vi "Read ADU Packet.vi"(8 "error in":errorcluster, 10 "Network Protocol":refnum<class "Network Protocol.lvclass">, 11 "ASCII transmission data unit in":refnum<class "ASCII Data Unit.lvclass">) -> (0 "error out":errorcluster, 1 "modbus data unit":refnum<class "Modbus Data Unit (PDU).lvclass">, 2 "Network Protocol out":refnum<class "Network Protocol.lvclass">, 3 "ASCII transmission data unit out":refnum<class "ASCII Data Unit.lvclass">, 5 "PDU Valid?":bool)   [LabVIEW 2020, in "SubVIs.lvlib" / "ASCII Data Unit.lvclass"]
uses:
  <vilib>/Modbus/subvis/Transmission Data Unit (ADU)/ASCII Data Unit/ASCII Data Unit.lvclass
  C:/builds/penguin/iak/lvdsc/trunk/20.0/lv/vi.lib/Modbus/subvis/Transmission Data Unit (ADU)/Transmission Data Unit/Transmission Data Unit.lvclass
  <vilib>/Modbus/subvis/Modbus Data Unit (PDU)/Modbus Data Unit (PDU).lvclass
  <vilib>/Modbus/subvis/Protocol/Interfaces/Network Protocol/Network Protocol.lvclass
  <vilib>/Modbus/subvis/Protocol/Serial/Serial Slave/Serial Slave.lvclass
  <vilib>/Modbus/subvis/Protocol/Serial/Serial Slave/Serial Slave.lvclass/Serial Slave.ctl
  <vilib>/Modbus/subvis/Protocol/Serial/Serial Master/Serial Master.lvclass
  <vilib>/Modbus/subvis/Protocol/Serial/Serial Master/Serial Master.lvclass/Serial Master.ctl
  <vilib>/Modbus/subvis/Transmission Data Unit (ADU)/Transmission Data Unit/Transmission Data Unit.lvclass/Transmission Data Unit.ctl
  <vilib>/Modbus/subvis/Modbus Data Unit (PDU)/Modbus Data Unit (PDU).lvclass/Modbus Data Unit (PDU).ctl
  <vilib>/Modbus/subvis/Transmission Data Unit (ADU)/ASCII Data Unit/ASCII Data Unit.lvclass/ASCII Data Unit.ctl
  <vilib>/ErrorRing/Error Ring.xnode
  <vilib>/Modbus/subvis/Transmission Data Unit (ADU)/Transmission Data Unit/Transmission Data Unit.lvclass
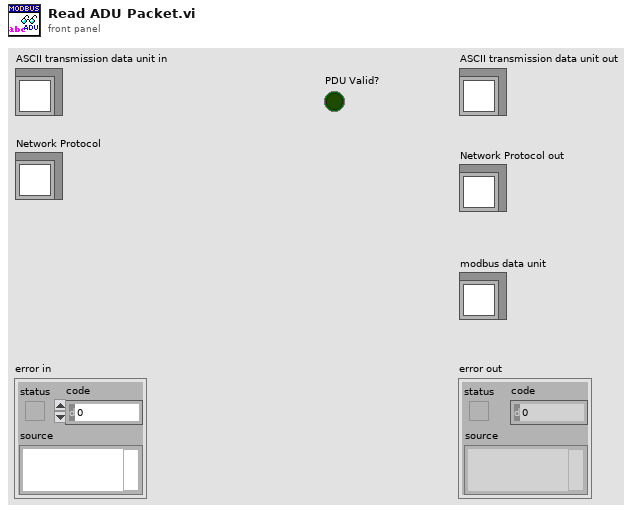
[diagram p1: front panel]
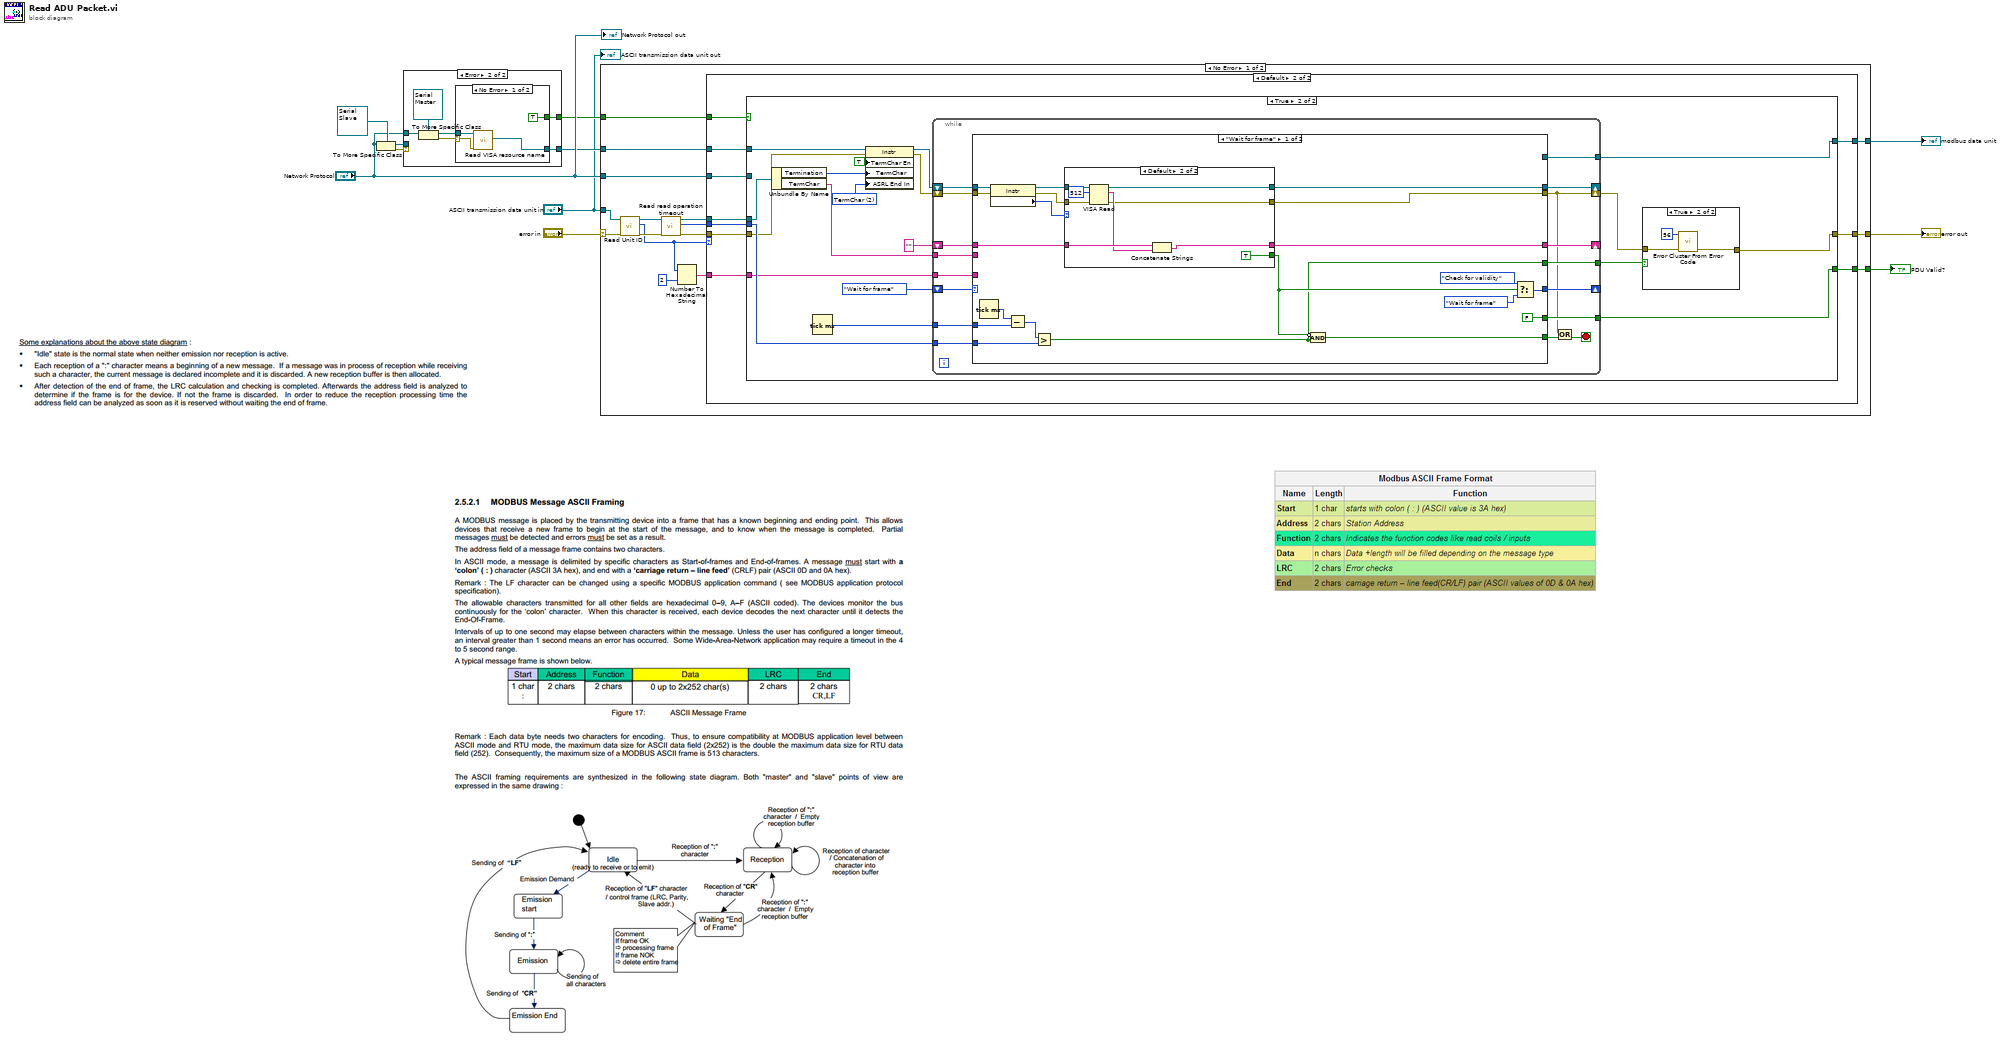
[diagram p0: block diagram]
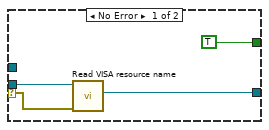
[diagram p2: hidden frame]
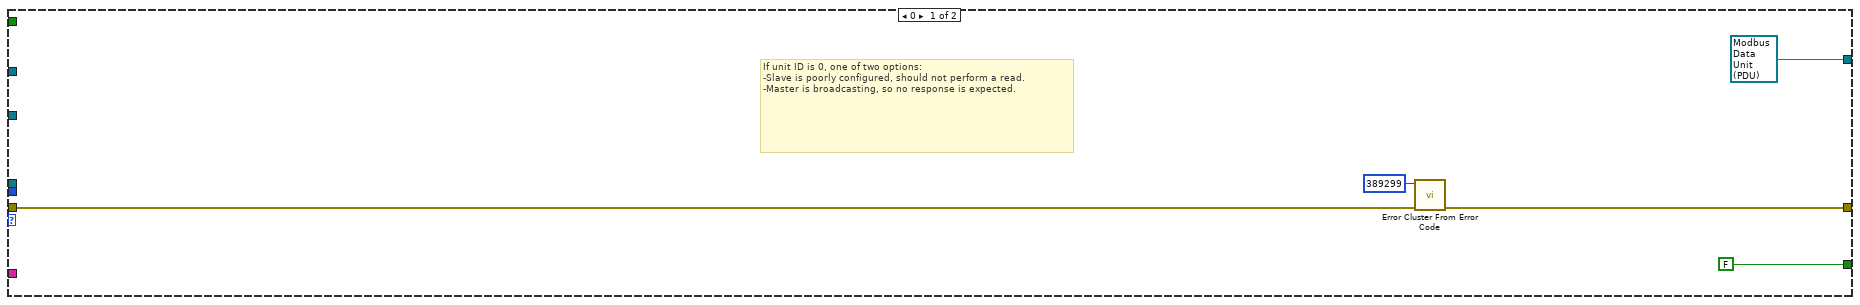
[diagram p4: hidden frame]
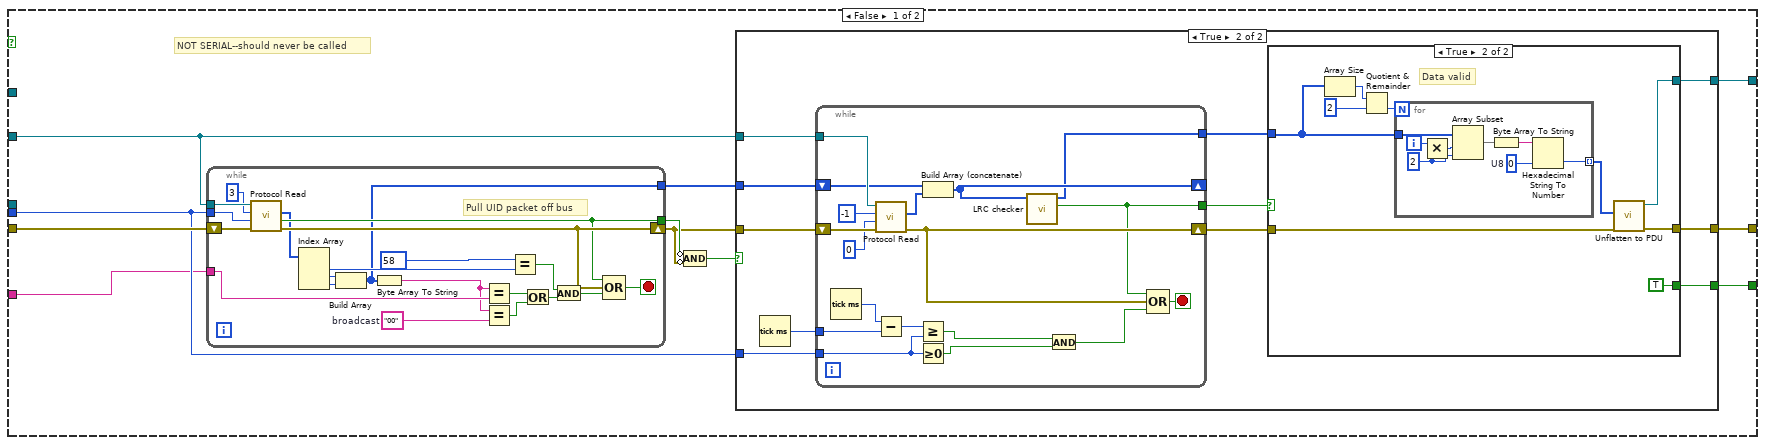
[diagram p5: hidden frame]
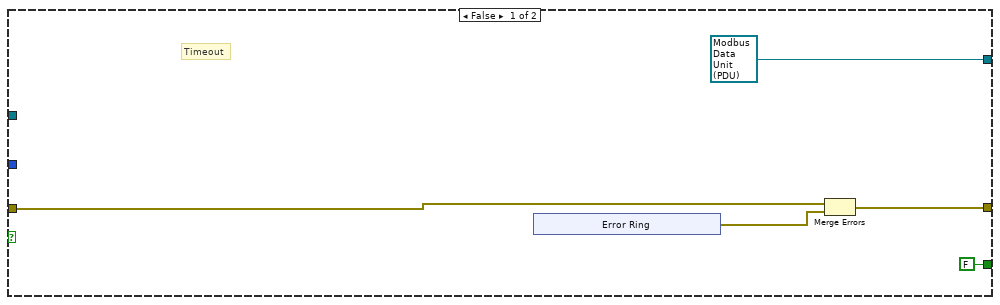
[diagram p6: hidden frame]
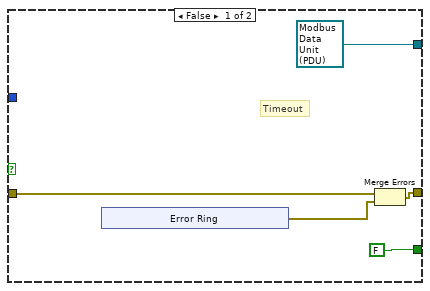
[diagram p7: hidden frame]
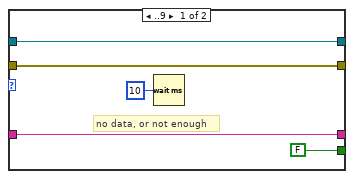
[diagram p9: hidden frame]
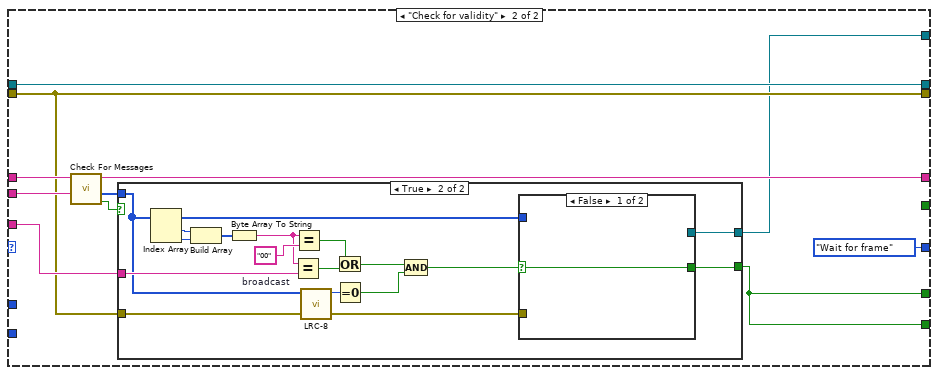
[diagram p10: hidden frame]
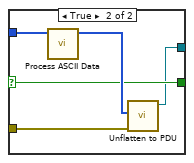
[diagram p12: hidden frame]
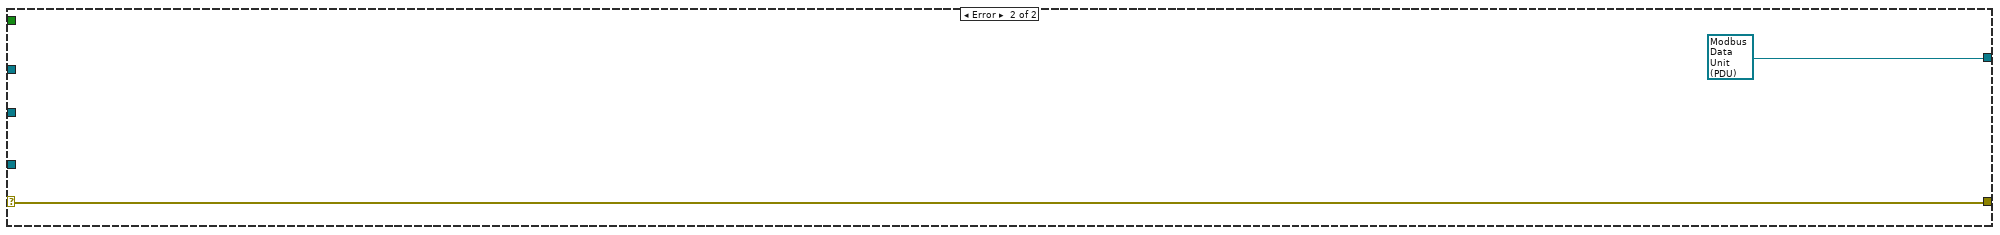
[diagram p13: hidden frame]
diagram:
  n1 = To More Specific Class(target class=refnum<class "Serial Slave.lvclass"> refnum ("Serial Master"), reference="Network Protocol") -> (specific class reference=w3:refnum<class "Serial Slave.lvclass">, error out=w6:errorcluster)  [unwired: 1 in]
  n2 = case shown="Error" w6 {
    selector: w6 -> [w13 _]
    tunnel: "Network Protocol" -> [_ w21]
    tunnel: [TRUE w18] -> w4
    tunnel: w3 -> [w14 _]
    tunnel: [w12 w16] -> w2
    frame No Error {
      n3 = call <vilib>:"Read VISA resource name.vi"("error in (no error)"=w13, "serial slave in"=w14) -> ("VISA resource name"=w12:refnum<visa-resource-name>)  [unwired: 7 in, 2 out]
    }
    frame Error {
      n4 = To More Specific Class(target class=refnum<class "Serial Master.lvclass"> refnum ("Serial Slave"), reference=w21) -> (specific class reference=w17:refnum<class "Serial Master.lvclass">, error out=w19:errorcluster)  [unwired: 1 in]
      n5 = case shown="No Error" w19 {
        selector: w19 -> [w23 _]
        tunnel: [TRUE _] -> w18
        tunnel: w17 -> [w24 _]
        tunnel: [w22 _] -> w16
        frame No Error {
          n6 = call <vilib>:"Read VISA resource name.vi"("error in (no error)"=w23, "serial master in"=w24) -> ("VISA resource name"=w22:refnum<visa-resource-name>)  [unwired: 7 in, 2 out]
        }
        frame Error {
        }
      }
    }
  }
  n7 = case shown="No Error" "error in" {
    selector: "error in" -> [w37 w262]
    tunnel: [w41 w262] -> w9
    tunnel: "ASCII transmission data unit in" -> [w27 _]
    tunnel: "Network Protocol" -> [w39 _]
    tunnel: [w40 refnum<class "Modbus Data Unit (PDU).lvclass"> refnum ("modbus data unit")] -> w10
    tunnel: [w33 _] -> w8
    tunnel: w4 -> [w32 _]
    tunnel: w2 -> [w28 _]
    frame No Error {
      n8 = call <vilib>:"Read Unit ID.vi"("error in"=w37, "transmission data unit in"=w27) -> ("error out"=w36:errorcluster, "unit ID"=w30:u8, "transmission data unit out"=w38:refnum<class "ASCII Data Unit.lvclass">)  [unwired: 7 in]
      n9 = call <vilib>:"Read read operation timeout.vi"("error in (no error)"=w36, "transmission data unit in"=w38) -> ("error out"=w35:errorcluster, "read operation timeout"=w34:i32, "transmission data unit out"=w26:refnum<class "ASCII Data Unit.lvclass">)  [unwired: 7 in]
      n10 = Number To Hexadecimal String(1:i16 2 ("width (-)"), 2:w30) -> (0:w29:string)
      n11 = case shown="Default" w30 {
        tunnel: w35 -> [w46 w52]
        tunnel: [w43 w56] -> w41
        tunnel: [refnum<class "Modbus Data Unit (PDU).lvclass"> refnum ("modbus data unit out") w55] -> w40
        tunnel: w39 -> [_ w51]
        tunnel: w34 -> [_ w54]
        tunnel: [FALSE w53] -> w33
        tunnel: w32 -> [_ w50]
        tunnel: w29 -> [_ w49]
        tunnel: w28 -> [_ w48]
        tunnel: w26 -> [_ w47]
        frame 0 {
          # "If unit ID is 0, one of two options:\n-Slave is poorly configured, should not perform a read.\n-Master is broadcasting, so no response is expected."
          n12 = call <vilib>:"Error Cluster From Error Code.vi"("error in (no error)"=w46, "error code (0)"=389299) -> ("error out"=w43:errorcluster)  [unwired: 7 in]
        }
        frame Default {
          n13 = case shown="True" w50 {
            tunnel: w52 -> [w67 w161]
            tunnel: [w63 w155] -> w56
            tunnel: [w62 w154] -> w55
            tunnel: w51 -> [w61 _]
            tunnel: w54 -> [w59 w162]
            tunnel: [w58 w160] -> w53
            tunnel: w49 -> [w57 w158]
            tunnel: w48 -> [_ w169]
            tunnel: w47 -> [_ w153]
            frame False {
              # "NOT SERIAL--should never be called"
              n14 = while {
                shift-right: [w149] -> w64
                shift-left: w67 -> [w152]
                tunnel: w59 -> [w147]
                tunnel: [w145] -> w66
                tunnel: [w137] -> w60
                tunnel: w61 -> [w151]
                tunnel: w57 -> [w138]
                stop <- w150 stop-if-true
                w132 = "00"  # broadcast
                # "Pull UID packet off bus"
                n15 = call-dynamic "Protocol Read.vi"("error in (no error)"=w152, "timeout"=w147, "bytes to read"=3, "protocol layer in"=w151) -> ("error out"=w149:errorcluster, "timed out?"=w145:bool, "data"=w144:u8[])  [unwired: 4 in, 1 out]
                n16 = Index Array(array=w144) -> (element #1=w142:u8, element #2=w140:u8, element #3=w139:u8)  [unwired: 3 in]
                n17 = Build Array(w140, w139) -> (w137:u8[])
                n18 = Byte Array To String(unsigned byte array=w137) -> (string=w133:string)
                n19 = Equal?(x=w133, y=w138) -> (x = y?=w135:bool)
                n20 = Equal?(x=w133, y=w132) -> (x = y?=w134:bool)
                n21 = Equal?(x=u8 58 ("y"), y=w142) -> (x = y?=w141:bool)
                n22 = Or(x=w135, y=w134) -> (x .or. y?=w136:bool)
                n23 = And(x=w141, y=w136) -> (x .and. y?=w146:bool)
                n24 = Compound Arithmetic op=OR(w145, w149, w146) -> (w150:bool)
              }
              n25 = Compound Arithmetic op=AND(invert w66, invert w64) -> (w65:bool)
              n26 = case shown="True" w65 {
                tunnel: w64 -> [w70 w87]
                tunnel: [w71 w79] -> w63
                tunnel: [refnum<class "Modbus Data Unit (PDU).lvclass"> refnum ("modbus data unit out") w80] -> w62
                tunnel: w61 -> [_ w83]
                tunnel: w60 -> [_ w84]
                tunnel: w59 -> [_ w85]
                tunnel: [FALSE w77] -> w58
                frame False {
                  # "Timeout"
                  n27 = xnode "Error Ring"() -> ("error out"=w72:errorcluster)
                  n28 = Merge Errors(w70, w72) -> (w71:errorcluster)
                }
                frame True {
                  n29 = Tick Count (ms)() -> (millisecond timer value=w86:u32)
                  n30 = while {
                    shift-right: [w117] -> w81
                    shift-left: w87 -> [w123]
                    tunnel: w86 -> [w131]
                    tunnel: w85 -> [w128]
                    shift-right: [w116] -> _
                    shift-left: w84 -> [w119]
                    tunnel: w83 -> [w122]
                    tunnel: [w114] -> w82
                    tunnel: [w115] -> w78
                    stop <- w125 stop-if-true
                    n31 = Tick Count (ms)() -> (millisecond timer value=w130:u32)
                    n32 = call-dynamic "Protocol Read.vi"("error in (no error)"=w123, "timeout"=0, "bytes to read"=-1, "protocol layer in"=w122) -> ("error out"=w117:errorcluster, "data"=w118:u8[])  [unwired: 4 in, 2 out]
                    n33 = Subtract(x=w130, y=w131) -> (x-y=w129:u32)
                    n34 = Greater Or Equal?(x=w129, y=w128) -> (x >= y?=w126:bool)
                    n35 = Greater Or Equal To 0?(x=w128) -> (x >= 0?=w127:bool)
                    n36 = Build Array (concatenate)(w119, w118) -> (w116:u8[])
                    n37 = call <vilib>:"LRC checker.vi"("data in"=w116) -> ("valid?"=w114:bool, "function data out"=w115:u8[])  [unwired: 9 in]
                    n38 = And(x=w126, y=w127) -> (x .and. y?=w124:bool)
                    n39 = Compound Arithmetic op=OR(w114, w117, w124) -> (w125:bool)
                  }
                  n40 = case shown="True" w82 {
                    tunnel: w81 -> [w90 w103]
                    tunnel: [refnum<class "Modbus Data Unit (PDU).lvclass"> refnum ("modbus data unit") w104] -> w80
                    tunnel: [w89 w105] -> w79
                    tunnel: w78 -> [_ w98]
                    tunnel: [FALSE TRUE] -> w77
                    frame False {
                      # "Timeout"
                      n41 = xnode "Error Ring"() -> ("error out"=w91:errorcluster)
                      n42 = Merge Errors(w90, w91) -> (w89:errorcluster)
                    }
                    frame True {
                      # "Data valid"
                      n43 = Array Size(array=w98) -> (size(s)=w102:i32)
                      n44 = Quotient & Remainder(x=w102, y=2) -> (floor(x/y)=w100:i32)  [unwired: 1 out]
                      n45 = for {
                        N: w100 -> [_]
                        tunnel: w98 -> [w113]
                        tunnel: [w106] -> w99 mode=indexing
                        i -> [w112]
                        w107 = u8 0  # U8
                        w111 = 2 ("length")
                        n46 = Multiply(x=w112, y=w111) -> (x*y=w110:i32)
                        n47 = Array Subset(array=w113, index=w110, length=w111) -> (w109:u8[])
                        n48 = Byte Array To String(unsigned byte array=w109) -> (string=w108:string)
                        n49 = Hexadecimal String To Number(string=w108, default (0uL)=w107) -> (number=w106:u8)  [unwired: 2 out]
                      }
                      n50 = call <vilib>:"Unflatten to PDU.vi"("error in (no error)"=w103, "Modbus data unit data"=w99) -> ("error out"=w105:errorcluster, "Modbus data unit out"=w104:refnum<class "Modbus Data Unit (PDU).lvclass">)  [unwired: 8 in]
                    }
                  }
                }
              }
            }
            frame True {
              w170 = u16 2 items=["None", "Last Bit", "TermChar"] ("Serial Settings:End Mode for Reads")
              n51 = Unbundle By Name(w153) -> ("Termination"=w168:u8, "TermChar"=w159:string)
              n52 = Tick Count (ms)() -> (millisecond timer value=w163:u32)
              n53 = property class="Instr"(reference=w169, error in=w161, "TermChar En"=TRUE ("Message Based Settings:Termination Character Enable"), "TermChar"=w168, "ASRL End In"=w170) -> (reference out=w166:refnum<visa-resource-name>, error out=w165:errorcluster)
              n54 = while {
                shift-right: [w191] -> _
                shift-left: enum16{"Wait for frame", "Check for validity"}."Wait for frame" ("Serial Acquisition States") -> [w192]
                shift-right: [w176] -> w156
                shift-left: w165 -> [w189]
                shift-right: [w183] -> _
                shift-left: w166 -> [w190]
                shift-right: [w187] -> _
                shift-left: "" -> [w188]
                tunnel: w163 -> [w186]
                tunnel: w162 -> [w185]
                tunnel: [w182] -> w160
                tunnel: w159 -> [w181]
                tunnel: w158 -> [w180]
                tunnel: [w179] -> w157
                tunnel: [w178] -> w154
                stop <- w177 stop-if-true
                n55 = case shown="\"Wait for frame\"" w192 {
                  tunnel: [w212 enum16{"Wait for frame", "Check for validity"}."Wait for frame" ("Serial Acquisition States")] -> w191
                  tunnel: w190 -> [w207 w236]
                  tunnel: w189 -> [w206 w229]
                  tunnel: w188 -> [w205 w235]
                  tunnel: [w204 w233] -> w187
                  tunnel: w186 -> [w202 _]
                  tunnel: w185 -> [w200 _]
                  tunnel: [w195 w228] -> w184
                  tunnel: [w197 w229] -> w176
                  tunnel: [w196 w236] -> w183
                  tunnel: [FALSE w228] -> w182
                  tunnel: w181 -> [_ w234]
                  tunnel: w180 -> [_ w231]
                  tunnel: [w193 _] -> w179
                  tunnel: [_ w227] -> w178
                  frame "Wait for frame" {
                    n56 = Tick Count (ms)() -> (millisecond timer value=w203:u32)
                    n57 = property class="Instr"(reference=w207, error in=w206) -> (reference out=w209:refnum<visa-resource-name>, error out=w198:errorcluster, "Serial Settings:Number of Bytes at Serial Port"=w208:u32)
                    n58 = Subtract(x=w203, y=w202) -> (x-y=w201:u32)
                    n59 = Greater?(x=w201, y=w200) -> (0:w193:bool)
                    n60 = case shown="Default" w208 {
                      tunnel: w209 -> [w213 w226]
                      tunnel: w205 -> [w216 w225]
                      tunnel: [w216 w223] -> w204
                      tunnel: [FALSE TRUE] -> w199
                      tunnel: w198 -> [w214 w221]
                      tunnel: [w214 w220] -> w197
                      tunnel: [w213 w219] -> w196
                      frame ..9 {
                        # "no data, or not enough"
                        n61 = Wait (ms)(milliseconds to wait=u32 10) -> ()  [unwired: 1 out]
                      }
                      frame Default {
                        n62 = VISA Read(VISA resource name=w226, byte count=u32 512, error in (no error)=w221) -> (VISA resource name out=w219:refnum<visa-resource-name>, read buffer=w224:string, error out=w220:errorcluster)  [unwired: 1 out]
                        n63 = Concatenate Strings(w225, w224) -> (w223:string)
                      }
                    }
                    n64 = Compound Arithmetic op=AND(invert w199, w193) -> (w195:bool)
                    n65 = Select(t=enum16{"Wait for frame", "Check for validity"}."Check for validity" ("Serial Acquisition States"), s=w199, f=enum16{"Wait for frame", "Check for validity"}."Wait for frame" ("Serial Acquisition States")) -> (s? t:f=w212:enum16{"Wait for frame", "Check for validity"})
                  }
                  frame "Check for validity" {
                    n66 = call <vilib>:"Check For Messages.vi"("Term Char"=w234, "Input String"=w235) -> ("found?"=w230:bool, "data"=w232:u8[], "Remaining String"=w233:string)  [unwired: 7 in]
                    n67 = case shown="True" w230 {
                      selector: w230 -> [w238 _]
                      tunnel: w232 -> [_ w242]
                      tunnel: w231 -> [_ w244]
                      tunnel: w229 -> [_ w241]
                      tunnel: [w238 w240] -> w228
                      tunnel: [_ w239] -> w227
                      frame False {
                      }
                      frame True {
                        w252 = "00"  # broadcast
                        n68 = Index Array(array=w242) -> (element #1=w248:u8, element #2=w249:u8)  [unwired: 2 in]
                        n69 = Build Array(w248, w249) -> (w247:u8[])
                        n70 = Byte Array To String(unsigned byte array=w247) -> (string=w251:string)
                        n71 = Equal?(x=w251, y=w244) -> (x = y?=w245:bool)
                        n72 = Equal?(x=w251, y=w252) -> (x = y?=w250:bool)
                        n73 = call <vilib>:"LRC-8.vi"("data"=w242) -> ("LRC-8"=w253:u8)  [unwired: 10 in]
                        n74 = Or(x=w250, y=w245) -> (x .or. y?=w246:bool)
                        n75 = Equal To 0?(x=w253) -> (x = 0?=w254:bool)
                        n76 = Compound Arithmetic op=AND(w246, w254) -> (w243:bool)
                        n77 = case shown="False" w243 {
                          selector: w243 -> [w255 w257]
                          tunnel: w242 -> [_ w260]
                          tunnel: w241 -> [_ w259]
                          tunnel: [w255 w257] -> w240
                          tunnel: [_ w256] -> w239
                          frame False {
                          }
                          frame True {
                            n78 = call <vilib>:"Process ASCII Data.vi"("data"=w260) -> ("pdu"=w258:u8[])  [unwired: 10 in]
                            n79 = call <vilib>:"Unflatten to PDU.vi"("error in (no error)"=w259, "Modbus data unit data"=w258) -> ("Modbus data unit out"=w256:refnum<class "Modbus Data Unit (PDU).lvclass">)  [unwired: 8 in, 1 out]
                          }
                        }
                      }
                    }
                  }
                }
                n80 = Or(x=w176, y=w184) -> (x .or. y?=w177:bool)
              }
              n81 = case shown="True" w157 {
                tunnel: w156 -> [w172 w175]
                tunnel: [w172 w173] -> w155
                frame False {
                }
                frame True {
                  n82 = call <vilib>:"Error Cluster From Error Code.vi"("error in (no error)"=w175, "error code (0)"=56) -> ("error out"=w173:errorcluster)  [unwired: 7 in]
                }
              }
            }
          }
        }
      }
    }
    frame Error {
    }
  }
  "modbus data unit" <- w10
  "error out" <- w9
  "PDU Valid?" <- w8
  "ASCII transmission data unit out" <- "ASCII transmission data unit in"
  "Network Protocol out" <- "Network Protocol"
